vi "Process-Next.vi"(8 "error in (no error)":errorcluster, 10 "Parameters":refnum<vi>, 11 "Process in":refnum<vi>) -> (0 "error out":errorcluster)   [LabVIEW 2016]
uses:
  controls/Parameters.ctl
  controls/Lambda.ctl
  <vilib>/Analysis/NI_AALBase.lvlib
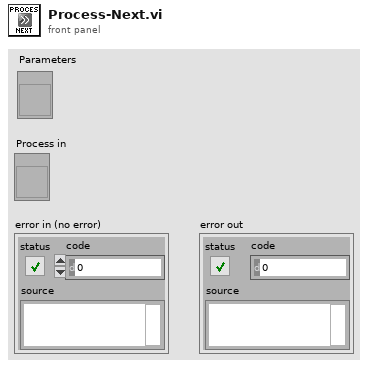
[diagram p1: front panel]
types:
  T1 = typedef "Parameters.ctl" = cluster{"Lambda":T2, "Power":dbl, "Frequency":dbl, "Stabilizing":dbl, "Samples":dbl, "File":path}
  T2 = typedef "Lambda.ctl" = cluster{"Init":dbl, "Final":dbl, "dx":dbl}
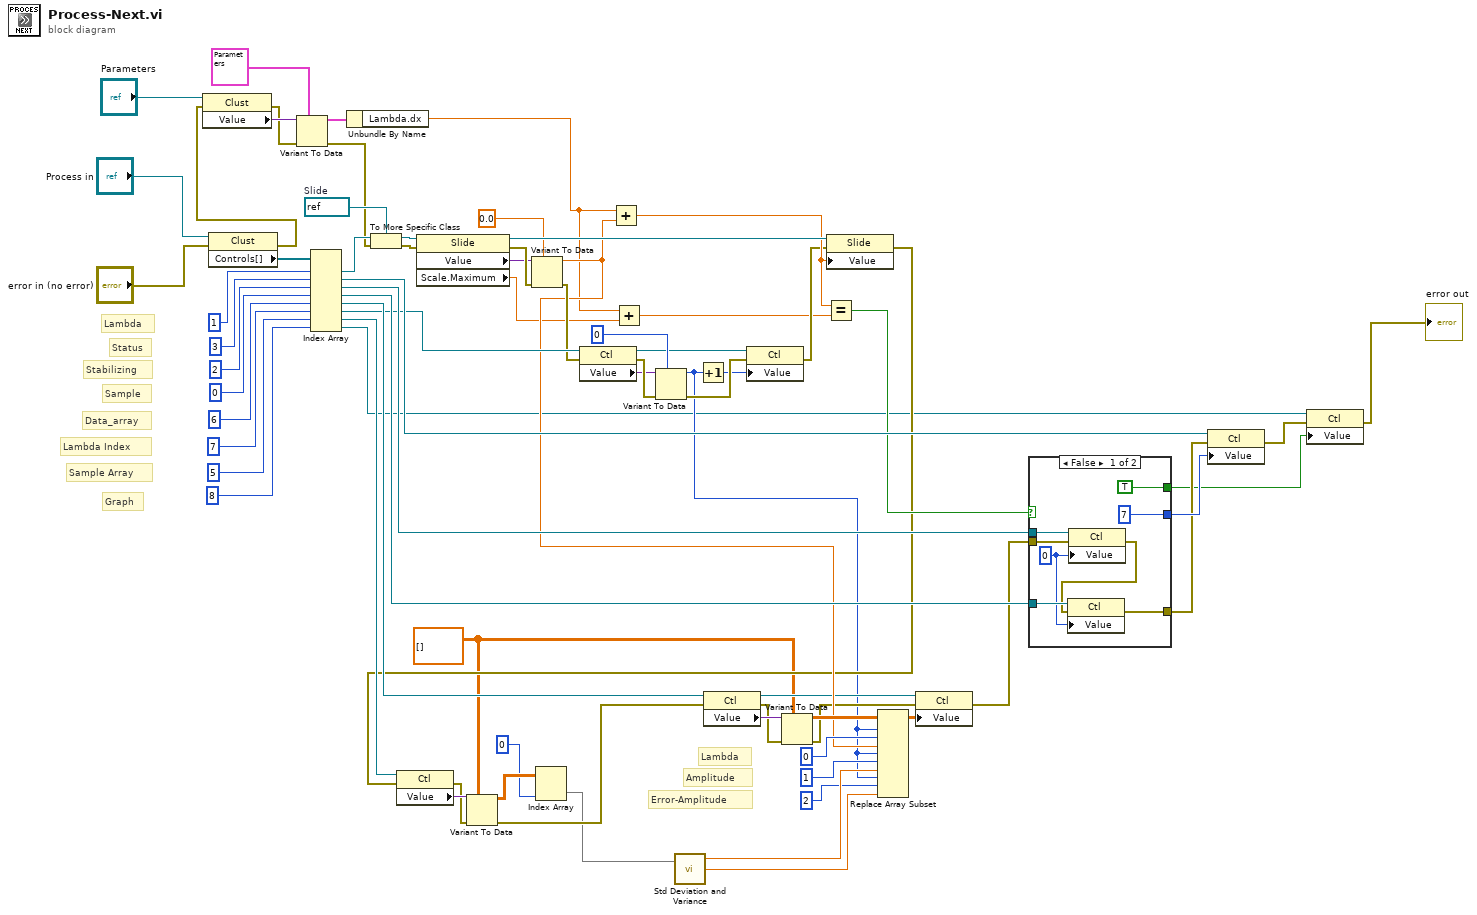
[diagram p0: block diagram]
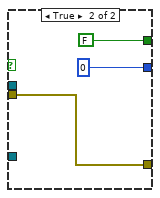
[diagram p2: hidden frame]
diagram:
  w17 = dbl[][] []
  w67 = refnum<vi> refnum  # Slide
  # "Graph"
  # "Error-Amplitude"
  # "Sample Array"
  # "Amplitude"
  # "Lambda"
  # "Lambda Index"
  # "Data_array"
  # "Sample"
  # "Stabilizing"
  # "Status"
  # "Lambda"
  n1 = property class="Clust"(reference="Process in", error in="error in (no error)") -> (error out=w49:errorcluster, "Controls[]"=w64:refnum<vi>[])  [unwired: 1 out]
  n2 = property class="Clust"(reference="Parameters", error in=w49) -> (error out=w47:errorcluster, "Value"=w48:variant)  [unwired: 1 out]
  n3 = Variant To Data(error in=w47, type=T1 {"Lambda"={"Init"=0.0, "Final"=0.0, "dx"=0.0}, "Power"=0.0, "Frequency"=0.0, "Stabilizing"=0.0, "Samples"=0.0, "File"=path ""} ("Parameters"), Variant=w48) -> (data=w44:T1, error out=w45:errorcluster)
  n4 = Index Array(array=w64, index #1=1 ("index"), index #2=3 ("index"), index #3=2 ("index"), index #4=0 ("index"), index #5=6, index #6=7 ("index"), index #7=5, index #8=8 ("index")) -> (element #1=w66:refnum<vi>, element #2=w61:refnum<vi>, element #3=w56:refnum<vi>, element #4=w54:refnum<vi>, element #5=w43:refnum<vi>, element #6=w39:refnum<vi>, element #7=w21:refnum<vi>, element #8=w3:refnum<vi>)
  n5 = Unbundle By Name(w44) -> ("Lambda.dx"=w8:dbl)
  n6 = To More Specific Class(target class=w67, reference=w66, error in=w45) -> (specific class reference=w69:refnum<vi>, error out=w68:errorcluster)
  n7 = property class="Slide"(reference=w69, error in=w68) -> (reference out=w72:refnum<vi>, error out=w71:errorcluster, "Value"=w70:variant, "Scale.Maximum"=w7:dbl)
  n8 = Variant To Data(error in=w71, type=0.0, Variant=w70) -> (data=w28:dbl, error out=w32:errorcluster)
  n9 = property class="Ctl"(reference=w39, error in=w32) -> (reference out=w35:refnum<vi>, error out=w38:errorcluster, "Value"=w37:variant)
  n10 = Add(x=w8, y=w28) -> (x+y=w52:dbl)
  n11 = Add(x=w8, y=w7) -> (x+y=w6:dbl)
  n12 = Variant To Data(error in=w38, type=0, Variant=w37) -> (data=w11:i32, error out=w34:errorcluster)
  n13 = Increment(x=w11) -> (x+1=w33:i32)
  n14 = property class="Ctl"(reference=w35, error in=w34, "Value"=w33) -> (error out=w31:errorcluster)  [unwired: 1 out]
  n15 = Equal?(x=w52, y=w6) -> (x = y?=w58:bool)
  n16 = property class="Slide"(reference=w72, error in=w31, "Value"=w52) -> (error out=w20:errorcluster)  [unwired: 1 out]
  n17 = property class="Ctl"(reference=w21, error in=w20) -> (error out=w18:errorcluster, "Value"=w19:variant)  [unwired: 1 out]
  n18 = Variant To Data(error in=w18, type=w17, Variant=w19) -> (data=w15:dbl[][], error out=w16:errorcluster)
  n19 = Index Array(array=w15, index (col)=0 ("disabled index (col)")) -> (element=w13:dbl[])  [unwired: 1 in]
  n20 = call <vilib>:"Std Deviation and Variance.vi"("X"=w13) -> ("mean"=w12:dbl, "standard deviation"=w9:dbl)  [unwired: 1 in, 1 out]
  n21 = property class="Ctl"(reference=w43, error in=w16) -> (reference out=w27:refnum<vi>, error out=w41:errorcluster, "Value"=w42:variant)
  n22 = Variant To Data(error in=w41, type=w17, Variant=w42) -> (data=w30:dbl[][], error out=w25:errorcluster)
  n23 = Replace Array Subset(array=w30, new element #1=w28, index (row) #1=w11, index (col) #1=0 ("disabled index (col)"), new element #2=w12, index (row) #2=w11, index (col) #2=1 ("disabled index (col)"), new element #3=w9, index (row) #3=w11, index (col) #3=2) -> (w26:dbl[][])
  n24 = property class="Ctl"(reference=w27, error in=w25, "Value"=w26) -> (error out=w24:errorcluster)  [unwired: 1 out]
  n25 = case shown="False" w58 {
    tunnel: [7 0] -> w59
    tunnel: w24 -> [w80 w83]
    tunnel: w56 -> [w79 _]
    tunnel: w54 -> [w78 _]
    tunnel: [w76 w83] -> w53
    tunnel: [TRUE FALSE] -> w2
    frame False {
      w75 = 0
      n26 = property class="Ctl"(reference=w79, error in=w80, "Value"=w75) -> (error out=w77:errorcluster)  [unwired: 1 out]
      n27 = property class="Ctl"(reference=w78, error in=w77, "Value"=w75) -> (error out=w76:errorcluster)  [unwired: 1 out]
    }
    frame True {
    }
  }
  n28 = property class="Ctl"(reference=w61, error in=w53, "Value"=w59) -> (error out=w4:errorcluster)  [unwired: 1 out]
  n29 = property class="Ctl"(reference=w3, error in=w4, "Value"=w2) -> (error out=→"error out":errorcluster)  [unwired: 1 out]
